vi "Controlword selection.vi"(11 "Controlword":T2) -> (1 "Control Word Data":u8[](array[numeric]), 2 "Controlword Out":T1, 3 "Controlword U16":u16, 5 "address":u16 format="%04x")   [LabVIEW 2016, in "IgusMotorDrive.lvclass"]
doc: "Converts the control word enumeration to an array of control world data\n\n<b>Copyright (C) 2018 Control Software Solutions Limited. All rights reserved. </b>"
uses:
  IgusMotorDrive.lvclass
  typedefs/Controlword--enum.ctl
  typedefs/Controlword--cluster.ctl
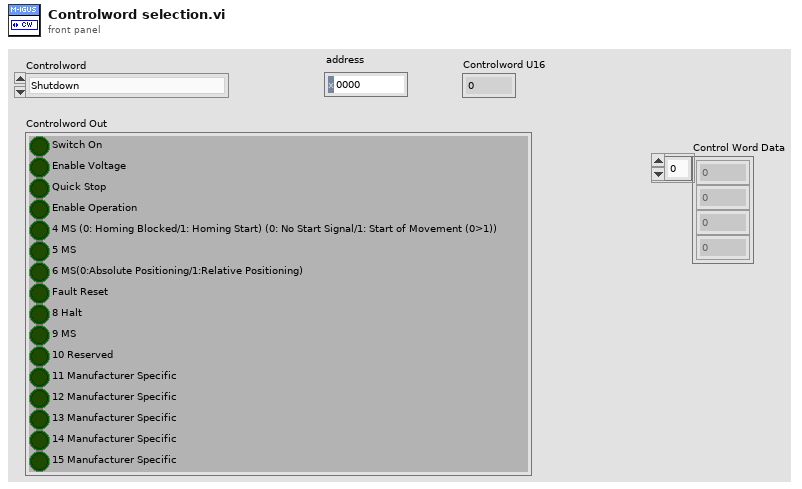
[diagram p1: front panel]
types:
  T1 = typedef "IgusMotorDrive.lvclass/Controlword--cluster.ctl" = cluster{"Switch On":bool, "Enable Voltage":bool, "Quick Stop":bool, "Enable Operation":bool, "4 MS (0: Homing Blocked/1: Homing Start) (0: No Start Signal/1: Start of Movement (0>1))":bool, "5 MS":bool, "6 MS(0:Absolute Positioning/1:Relative Positioning)":bool, "Fault Reset":bool, "8 Halt":bool, "9 MS":bool, "10 Reserved":bool, "11 Manufacturer Specific":bool, "12 Manufacturer Specific":bool, "13 Manufacturer Specific":bool, "14 Manufacturer Specific":bool, "15 Manufacturer Specific":bool}
  T2 = typedef "IgusMotorDrive.lvclass/Controlword--enum.ctl" = enum16{"Shutdown", "Switch On", "Switch On and Enable Operation", "Disable Voltage", "Halt", "Quick Stop", "Disable Operation", "Enable Operation", "Fault Reset"}
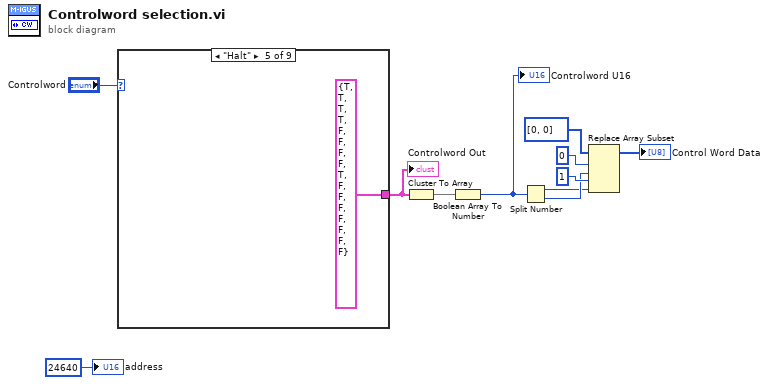
[diagram p0: block diagram]
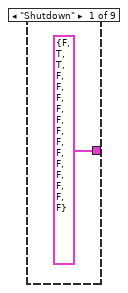
[diagram p2: hidden frame]
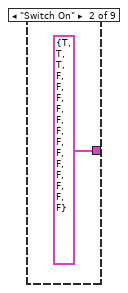
[diagram p3: hidden frame]
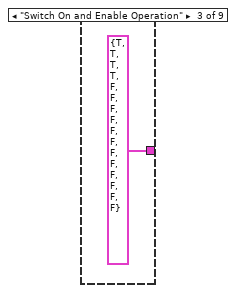
[diagram p4: hidden frame]
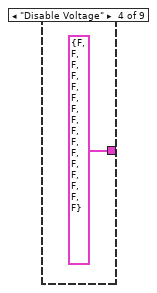
[diagram p5: hidden frame]
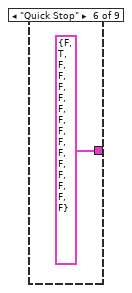
[diagram p6: hidden frame]
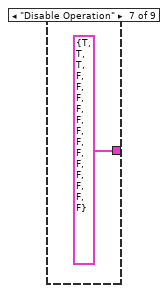
[diagram p7: hidden frame]
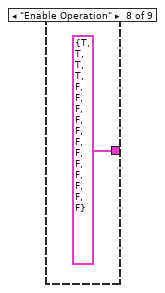
[diagram p8: hidden frame]
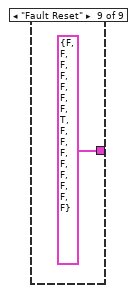
[diagram p9: hidden frame]
diagram:
  n1 = case shown="\"Halt\"" "Controlword" {
    tunnel: [T1 {"Switch On"=FALSE, "Enable Voltage"=TRUE, "Quick Stop"=TRUE, "Enable Operation"=FALSE, "4 MS (0: Homing Blocked/1: Homing Start) (0: No Start Signal/1: Start of Movement (0>1))"=FALSE, "5 MS"=FALSE, "6 MS(0:Absolute Positioning/1:Relative Positioning)"=FALSE, "Fault Reset"=FALSE, "8 Halt"=FALSE, "9 MS"=FALSE, "10 Reserved"=FALSE, "11 Manufacturer Specific"=FALSE, "12 Manufacturer Specific"=FALSE, "13 Manufacturer Specific"=FALSE, "14 Manufacturer Specific"=FALSE, "15 Manufacturer Specific"=FALSE} ("Controlword 2") T1 {"Switch On"=TRUE, "Enable Voltage"=TRUE, "Quick Stop"=TRUE, "Enable Operation"=FALSE, "4 MS (0: Homing Blocked/1: Homing Start) (0: No Start Signal/1: Start of Movement (0>1))"=FALSE, "5 MS"=FALSE, "6 MS(0:Absolute Positioning/1:Relative Positioning)"=FALSE, "Fault Reset"=FALSE, "8 Halt"=FALSE, "9 MS"=FALSE, "10 Reserved"=FALSE, "11 Manufacturer Specific"=FALSE, "12 Manufacturer Specific"=FALSE, "13 Manufacturer Specific"=FALSE, "14 Manufacturer Specific"=FALSE, "15 Manufacturer Specific"=FALSE} ("Controlword 2") T1 {"Switch On"=TRUE, "Enable Voltage"=TRUE, "Quick Stop"=TRUE, "Enable Operation"=TRUE, "4 MS (0: Homing Blocked/1: Homing Start) (0: No Start Signal/1: Start of Movement (0>1))"=FALSE, "5 MS"=FALSE, "6 MS(0:Absolute Positioning/1:Relative Positioning)"=FALSE, "Fault Reset"=FALSE, "8 Halt"=FALSE, "9 MS"=FALSE, "10 Reserved"=FALSE, "11 Manufacturer Specific"=FALSE, "12 Manufacturer Specific"=FALSE, "13 Manufacturer Specific"=FALSE, "14 Manufacturer Specific"=FALSE, "15 Manufacturer Specific"=FALSE} ("Controlword 2") T1 {"Switch On"=FALSE, "Enable Voltage"=FALSE, "Quick Stop"=FALSE, "Enable Operation"=FALSE, "4 MS (0: Homing Blocked/1: Homing Start) (0: No Start Signal/1: Start of Movement (0>1))"=FALSE, "5 MS"=FALSE, "6 MS(0:Absolute Positioning/1:Relative Positioning)"=FALSE, "Fault Reset"=FALSE, "8 Halt"=FALSE, "9 MS"=FALSE, "10 Reserved"=FALSE, "11 Manufacturer Specific"=FALSE, "12 Manufacturer Specific"=FALSE, "13 Manufacturer Specific"=FALSE, "14 Manufacturer Specific"=FALSE, "15 Manufacturer Specific"=FALSE} ("Controlword 2") T1 {"Switch On"=TRUE, "Enable Voltage"=TRUE, "Quick Stop"=TRUE, "Enable Operation"=TRUE, "4 MS (0: Homing Blocked/1: Homing Start) (0: No Start Signal/1: Start of Movement (0>1))"=FALSE, "5 MS"=FALSE, "6 MS(0:Absolute Positioning/1:Relative Positioning)"=FALSE, "Fault Reset"=FALSE, "8 Halt"=TRUE, "9 MS"=FALSE, "10 Reserved"=FALSE, "11 Manufacturer Specific"=FALSE, "12 Manufacturer Specific"=FALSE, "13 Manufacturer Specific"=FALSE, "14 Manufacturer Specific"=FALSE, "15 Manufacturer Specific"=FALSE} ("Controlword 2") T1 {"Switch On"=FALSE, "Enable Voltage"=TRUE, "Quick Stop"=FALSE, "Enable Operation"=FALSE, "4 MS (0: Homing Blocked/1: Homing Start) (0: No Start Signal/1: Start of Movement (0>1))"=FALSE, "5 MS"=FALSE, "6 MS(0:Absolute Positioning/1:Relative Positioning)"=FALSE, "Fault Reset"=FALSE, "8 Halt"=FALSE, "9 MS"=FALSE, "10 Reserved"=FALSE, "11 Manufacturer Specific"=FALSE, "12 Manufacturer Specific"=FALSE, "13 Manufacturer Specific"=FALSE, "14 Manufacturer Specific"=FALSE, "15 Manufacturer Specific"=FALSE} ("Controlword 2") T1 {"Switch On"=TRUE, "Enable Voltage"=TRUE, "Quick Stop"=TRUE, "Enable Operation"=FALSE, "4 MS (0: Homing Blocked/1: Homing Start) (0: No Start Signal/1: Start of Movement (0>1))"=FALSE, "5 MS"=FALSE, "6 MS(0:Absolute Positioning/1:Relative Positioning)"=FALSE, "Fault Reset"=FALSE, "8 Halt"=FALSE, "9 MS"=FALSE, "10 Reserved"=FALSE, "11 Manufacturer Specific"=FALSE, "12 Manufacturer Specific"=FALSE, "13 Manufacturer Specific"=FALSE, "14 Manufacturer Specific"=FALSE, "15 Manufacturer Specific"=FALSE} ("Controlword 2") T1 {"Switch On"=TRUE, "Enable Voltage"=TRUE, "Quick Stop"=TRUE, "Enable Operation"=TRUE, "4 MS (0: Homing Blocked/1: Homing Start) (0: No Start Signal/1: Start of Movement (0>1))"=FALSE, "5 MS"=FALSE, "6 MS(0:Absolute Positioning/1:Relative Positioning)"=FALSE, "Fault Reset"=FALSE, "8 Halt"=FALSE, "9 MS"=FALSE, "10 Reserved"=FALSE, "11 Manufacturer Specific"=FALSE, "12 Manufacturer Specific"=FALSE, "13 Manufacturer Specific"=FALSE, "14 Manufacturer Specific"=FALSE, "15 Manufacturer Specific"=FALSE} ("Controlword 2") T1 {"Switch On"=FALSE, "Enable Voltage"=FALSE, "Quick Stop"=FALSE, "Enable Operation"=FALSE, "4 MS (0: Homing Blocked/1: Homing Start) (0: No Start Signal/1: Start of Movement (0>1))"=FALSE, "5 MS"=FALSE, "6 MS(0:Absolute Positioning/1:Relative Positioning)"=FALSE, "Fault Reset"=TRUE, "8 Halt"=FALSE, "9 MS"=FALSE, "10 Reserved"=FALSE, "11 Manufacturer Specific"=FALSE, "12 Manufacturer Specific"=FALSE, "13 Manufacturer Specific"=FALSE, "14 Manufacturer Specific"=FALSE, "15 Manufacturer Specific"=FALSE} ("Controlword 2")] -> w10
    frame "Shutdown" {
    }
    frame "Switch On" {
    }
    frame "Switch On and Enable Operation" {
    }
    frame "Disable Voltage" {
    }
    frame "Halt" {
    }
    frame "Quick Stop" {
    }
    frame "Disable Operation" {
    }
    frame "Enable Operation" {
    }
    frame "Fault Reset" {
    }
  }
  "Controlword Out" <- w10
  n2 = Cluster To Array(cluster=w10) -> (array=w9:bool[])
  n3 = Boolean Array To Number(Boolean array=w9) -> (number=w2:u16)
  "Controlword U16" <- w2
  n4 = Split Number(x=w2) -> (hi(x)=w4:u8, lo(x)=w5:u8)
  n5 = Replace Array Subset(array=u8[] [0, 0] ("Data [1-4]"), new element #1=w5, index #1=0 ("index"), new element #2=w4, index #2=1 ("index")) -> (→"Control Word Data":u8[])
  "address" <- u16 24640 ("address")
